vi "Create Basic Measurement Annotations.vi"(8 "error in":errorcluster, 9 "tags":string[](array[string]), 10 "collection":string, 11 "description":string) -> (0 "error out":errorcluster, 3 "measurement annotations":T1[](array[typedef]))   [LabVIEW 2020, in "MeasurementLink Measurement Server.lvlib"]
uses:
  MeasurementLink Measurement Server.lvlib
  TypeDefs/Measurement Annotation.ctl
  a9ad9b04-f222-4ebf-94b5-602fd11bc15e.vi
  0221d297-ed52-46f4-bb7b-f2207ffca4d2.vi
  725c875f-b543-4029-b405-f80e7b23a3ec.vi
  e6ee6f9c-c471-4d22-be66-87c65b49d659.vi
  a9ad9b04-f222-4ebf-94b5-602fd11bc15e.vi/77476d48-7c31-46ad-92c1-ee98bcbcef06.vi
  0221d297-ed52-46f4-bb7b-f2207ffca4d2.vi/77476d48-7c31-46ad-92c1-ee98bcbcef06.vi
  725c875f-b543-4029-b405-f80e7b23a3ec.vi/77476d48-7c31-46ad-92c1-ee98bcbcef06.vi
  e6ee6f9c-c471-4d22-be66-87c65b49d659.vi/77476d48-7c31-46ad-92c1-ee98bcbcef06.vi
  <vilib>/Utility/Data Type/Get Type Information.vi
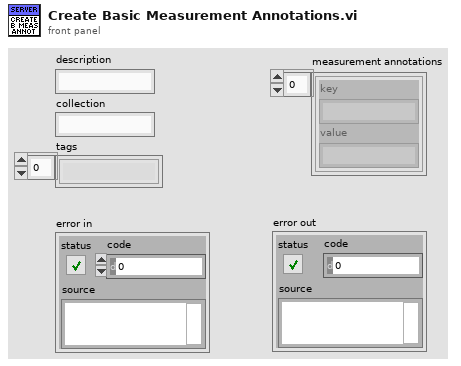
[diagram p1: front panel]
types:
  T1 = typedef "MeasurementLink Measurement Server.lvlib/Measurement Annotation.ctl" = cluster{"key":string, "value":string}
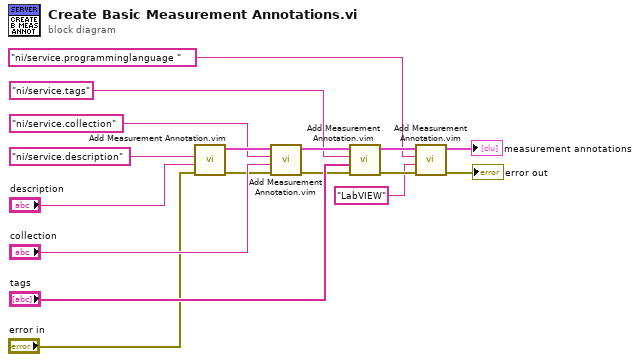
[diagram p0: block diagram]
diagram:
  n1 = call "Add Measurement Annotation.vim"("error in"="error in", "value (anything)"="description", "key"="ni/service.description" ("Key")) -> ("error out"=w8:errorcluster, "measurement annotations out"=w16:T1[])  [unwired: 7 in]
  n2 = call "Add Measurement Annotation.vim"("error in"=w8, "value (anything)"="collection", "key"="ni/service.collection" ("Key"), "measurement annotations in"=w16) -> ("error out"=w9:errorcluster, "measurement annotations out"=w17:T1[])  [unwired: 6 in]
  n3 = call "Add Measurement Annotation.vim"("error in"=w9, "value (anything)"="tags", "key"="ni/service.tags" ("Key"), "measurement annotations in"=w17) -> ("error out"=w6:errorcluster, "measurement annotations out"=w3:T1[])  [unwired: 6 in]
  n4 = call "Add Measurement Annotation.vim"("error in"=w6, "value (anything)"="LabVIEW", "key"="ni/service.programminglanguage " ("Key"), "measurement annotations in"=w3) -> ("error out"=→"error out":errorcluster, "measurement annotations out"=→"measurement annotations":T1[])  [unwired: 6 in]
